vi "Add_Update_Values_sub.vi"(5 "Raw data Filename column name":string, 6 "Edit all Rows?":bool, 7 "Value  Constant?":bool, 8 "Selected Rows":i32[](array[numeric]), 9 "New Values In":string[][](array[string]), 10 "New Chs In":string[](array[string])=[""], 11 "Filename":path) -> (1 "Edit Info":string[][](array[string]))   [LabVIEW 2021]
uses:
  Globals/Constants_global.vi
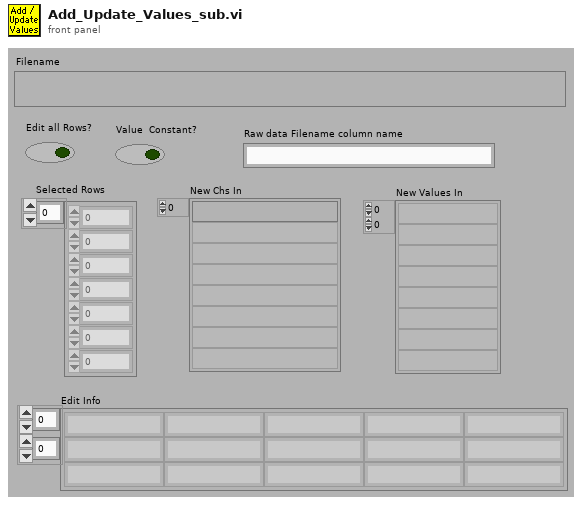
[diagram p1: front panel]
types:
  T1 = enum16{"read/write", "read-only", "write-only", "write-only (truncate)"}
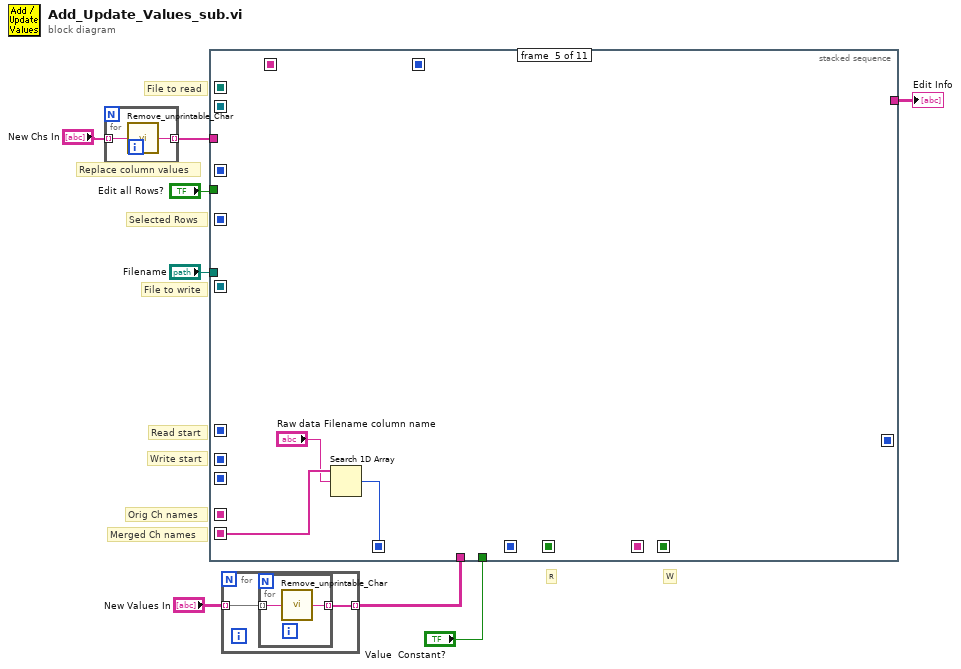
[diagram p0: block diagram]
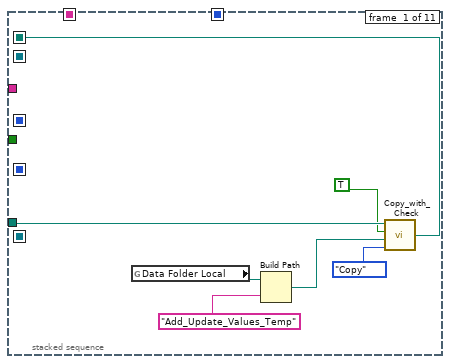
[diagram p2: hidden frame]
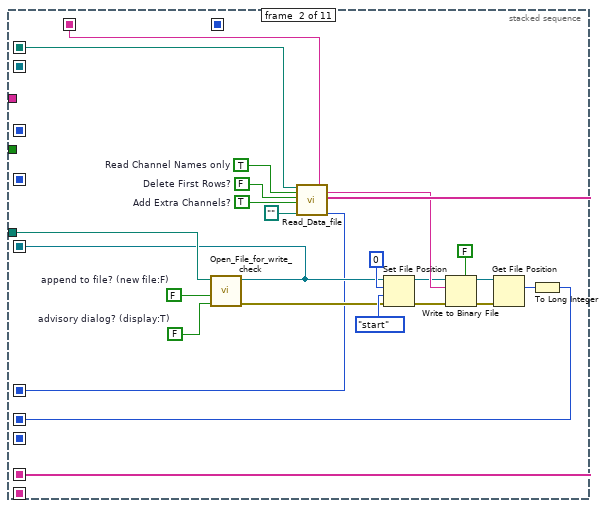
[diagram p3: hidden frame]
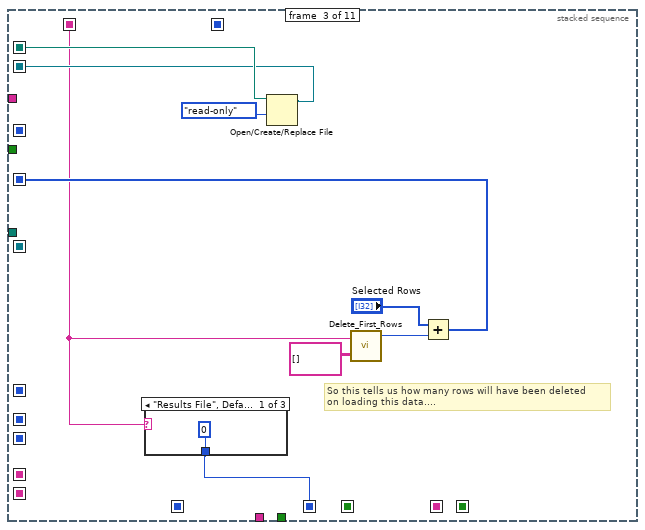
[diagram p4: hidden frame]
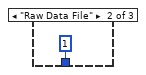
[diagram p5: hidden frame]
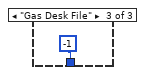
[diagram p6: hidden frame]
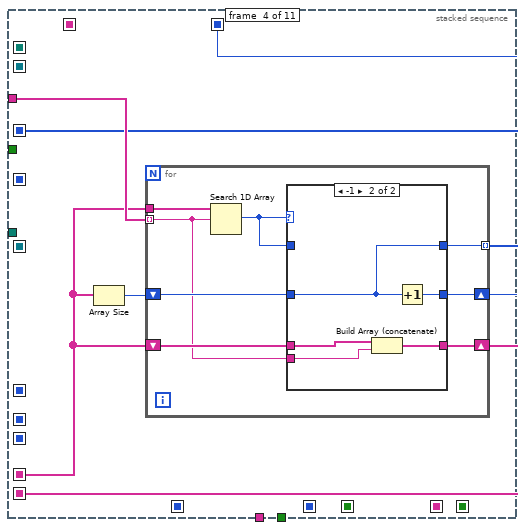
[diagram p7: hidden frame]
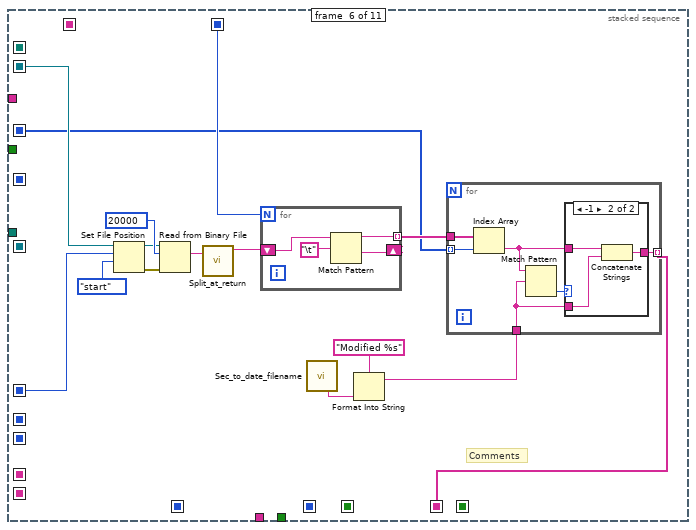
[diagram p9: hidden frame]
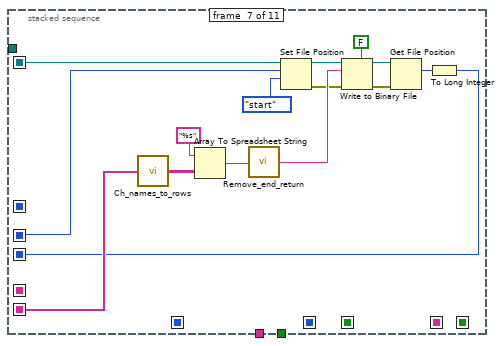
[diagram p11: hidden frame]
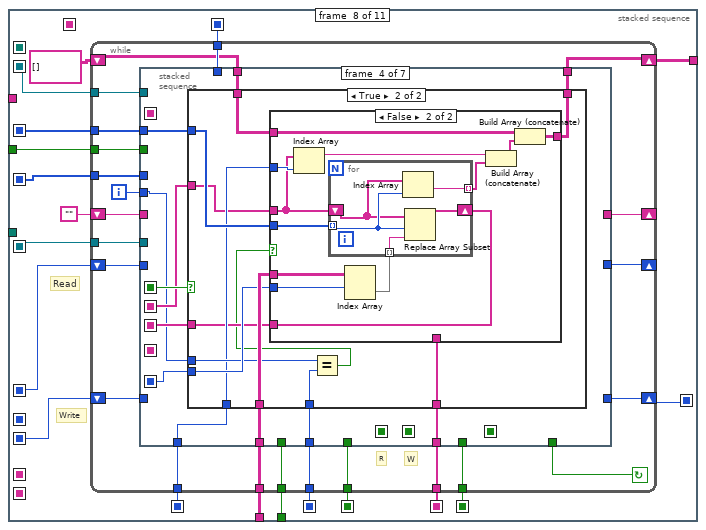
[diagram p12: hidden frame]
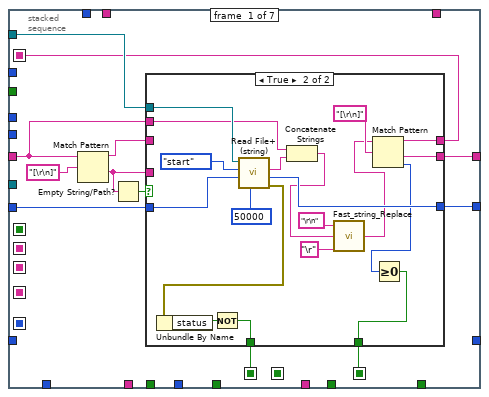
[diagram p13: hidden frame]
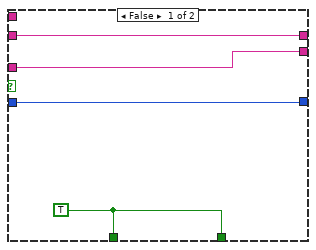
[diagram p14: hidden frame]
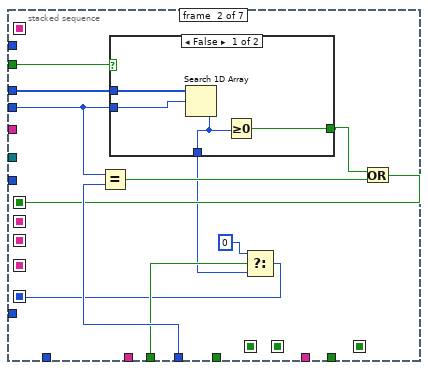
[diagram p15: hidden frame]
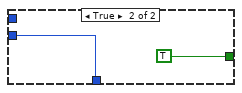
[diagram p16: hidden frame]
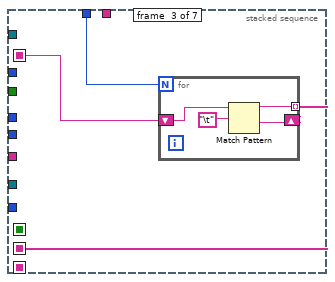
[diagram p17: hidden frame]
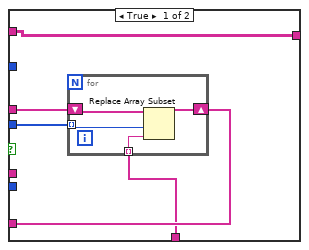
[diagram p19: hidden frame]
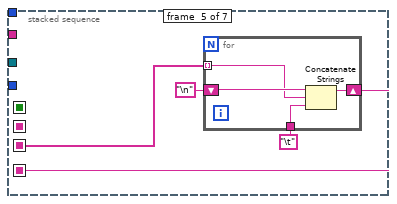
[diagram p20: hidden frame]
diagram:
  # "File to read"
  # "File to write"
  # "Merged Ch names"
  # "Orig Ch names"
  # "Replace column values"
  # "Selected Rows"
  # "Read start"
  # "Write start"
  # "W"
  # "R"
  n1 = for {
    tunnel: "New Chs In" -> [w10] mode=indexing
    tunnel: [w9] -> w4 mode=indexing
    n2 = call "Remove_unprintable_Char.vi"("Input String"=w10) -> ("Output String"=w9:string)
  }
  n3 = for {
    tunnel: "New Values In" -> [w12] mode=indexing
    tunnel: [w11] -> w2 mode=indexing
    n4 = for {
      tunnel: w12 -> [w14] mode=indexing
      tunnel: [w13] -> w11 mode=indexing
      n5 = call "Remove_unprintable_Char.vi"("Input String"=w14) -> ("Output String"=w13:string)
    }
  }
  n6 = stacked-sequence {
    seq-local: [_ _ w48 _ _ _ _ _ _ _ _] -> [_ _ _ _ _ w94 _ w137 _ w314 _]
    seq-local: [_ w31 _ _ _ _ _ _ _ _ _] -> [_ _ _ _ _ w93 _ w139 _ _ _]
    seq-local: [_ _ _ _ _ _ _ w143 _ _ _] -> [_ _ _ _ _ _ _ _ _ _ w318]
    seq-local: [_ _ _ _ _ _ _ w142 _ _ _] -> [_ _ _ _ _ _ _ _ _ _ w320]
    seq-local: [_ _ _ _ _ _ _ w141 _ _ _] -> [_ _ _ _ _ _ _ _ w311 _ _]
    seq-local: [_ _ w51 _ _ _ _ _ _ _ _] -> [_ _ _ _ _ _ _ w140 _ _ _]
    seq-local: [_ w32 _ _ _ _ _ _ _ _ _] -> [_ _ _ _ _ _ w119 _ _ _ _]
    seq-local: [_ w42 _ _ _ _ _ _ _ _ _] -> [_ _ _ w59 _ _ _ _ _ _ _]
    seq-local: [_ _ _ w60 _ _ _ _ _ _ _] -> [_ _ _ _ _ w88 _ w135 _ _ _]
    seq-local: [_ w34 _ _ _ _ _ _ _ _ _] -> [_ _ _ _ _ _ w120 w138 w309 w312 _]
    seq-local: [_ _ _ w58 _ _ _ _ _ _ _] -> [_ _ _ _ _ w96 _ w136 _ _ _]
    seq-local: [_ _ _ w57 _ _ _ _ _ _ _] -> [_ _ _ _ w81 _ w123 _ _ _ _]
    seq-local: [w16 _ _ _ _ _ _ _ _ _ _] -> [_ w41 w49 _ _ _ _ _ _ _ w316]
    seq-local: [_ _ _ _ _ _ w118 _ _ _ _] -> [_ _ _ _ _ _ _ w134 _ _ _]
    seq-local: [_ w30 _ _ _ _ _ _ _ _ _] -> [_ _ w46 _ _ _ _ _ _ _ _]
    seq-local: [_ _ _ _ _ w85 _ _ _ _ _] -> [_ _ _ _ _ _ _ w129 _ _ _]
    seq-local: [_ _ w47 _ _ _ _ _ _ _ _] -> [_ _ _ _ _ _ _ w130 _ _ _]
    seq-local: [_ _ _ _ w80 _ _ _ _ _ _] -> [_ _ _ _ _ _ _ w128 _ _ _]
    tunnel: "Filename" -> [w18 w35 _ _ _ _ _ _ _ _ w317]
    tunnel: w4 -> [_ _ _ w62 _ _ _ _ _ _ _]
    tunnel: "Edit all Rows?" -> [_ _ _ _ _ _ _ w133 _ _ _]
    tunnel: w2 -> [_ _ _ _ _ _ _ w132 _ _ _]
    tunnel: "Value  Constant?" -> [_ _ _ _ _ _ _ w131 _ _ _]
    tunnel: [_ _ _ _ _ _ _ w126 _ _ _] -> w5
    frame #0 {
      n7 = global read "Constants_global.vi" "Data Folder Local"() -> (w20:path)
      n8 = Build Path(base path=w20, name or relative path="Add_Update_Values_Temp") -> (appended path=w19:path)
      n9 = call "Copy_with_Check.vi"("Mode"=enum16{"Move", "Copy"}."Copy", "Target Path"=w19, "Variable Target?"=TRUE, "Source Path"=w18) -> ("Pathname Out"=w16:path)
    }
    frame #1 {
      w22 = FALSE  # Delete First Rows?
      w23 = TRUE  # Add Extra Channels?
      w39 = FALSE  # advisory dialog? (display:T)
      w40 = FALSE  # append to file? (new file:F)
      w43 = TRUE  # Read Channel Names only
      n10 = call "Open_File_for_write_check.vi"("advisory dialog? (display:T)"=w39, "append to file? (new file:F)"=w40, "file path"=w35) -> ("error out"=w36:errorcluster, "refnum"=w34:refnum<file>)  [unwired: 7 out]
      n11 = call "Read_Data_file.vi"("Results file"=w41, "Read Channel Names only"=w43, "Delete First Rows?"=w22, "Add Extra Channels?"=w23, "Template File"=path "") -> ("Filetype"=w30:string, "String Before"=w33:string, "Ch names Out"=w42:string[], "Start Bytes"=w31:i32)  [unwired: 2 in, 9 out]
      n12 = Set File Position(offset (in bytes) (0)=0 ("pos offset (0)"), refnum=w34, from (0:start)=enum16{"start", "end", "current"}."start" ("pos mode (0:2)"), error in=w36) -> (refnum out=w29:refnum<file>, error out=w28:errorcluster)
      n13 = Write to Binary File(file (use dialog)=w29, data=w33, error in=w28, 5:FALSE ("prepend array or string size? (T)")) -> (refnum out=w27:refnum<file>, error out=w26:errorcluster)  [unwired: 3 out]
      n14 = Get File Position(4:w26, 7:w27) -> (2:w25:i64)  [unwired: 2 out]
      n15 = To Long Integer(number=w25) -> (32bit integer=w32:i32)
    }
    frame #2 {
      # "So this tells us how many rows will have been deleted\non loading this data...."
      n16 = case shown="\"Results File\", Default" w46 {
        tunnel: [0 ("Comments Row Number") 1 ("Comments Row Number") -1 ("Comments Row Number")] -> w47
        frame "Results File", Default {
        }
        frame "Raw Data File" {
        }
        frame "Gas Desk File" {
        }
      }
      n17 = Open/Create/Replace File(file path (use dialog)=w49, access (0:read/write)=T1."read-only" ("open mode (0)")) -> (refnum out=w48:refnum<file>)  [unwired: 1 in, 5 out]
      n18 = call "Delete_First_Rows.vi"("File Type"=w46, "Data In"=string[][] []) -> ("Rows removed"=w53:i32)  [unwired: 2 out]
      n19 = Add(x="Selected Rows", y=w53) -> (x+y=w51:i32[])
    }
    frame #3 {
      n20 = Array Size(array=w59) -> (size(s)=w61:i32)
      n21 = for {
        tunnel: w59 -> [w70]
        tunnel: w62 -> [w63] mode=indexing
        shift-right: [w69] -> w58
        shift-left: w61 -> [w68]
        tunnel: [w67] -> w60 mode=indexing
        shift-right: [w64] -> w57
        shift-left: w59 -> [w65]
        n22 = Search 1D Array(1D array=w70, element=w63) -> (index of element=w66:i32)  [unwired: 1 out]
        n23 = case shown="-1" w66 {
          tunnel: [w72 w78] -> w69
          tunnel: w68 -> [w72 w77]
          tunnel: [w73 w77] -> w67
          tunnel: w66 -> [w73 _]
          tunnel: w65 -> [w71 w76]
          tunnel: [w71 w75] -> w64
          tunnel: w63 -> [_ w74]
          frame 0, Default {
          }
          frame -1 {
            n24 = Build Array (concatenate)(w76, w74) -> (w75:string[])
            n25 = Increment(x=w77) -> (x+1=w78:i32)
          }
        }
      }
    }
    frame #4 {
      n26 = Search 1D Array(1D array=w81, element="Raw data Filename column name") -> (index of element=w80:i32)  [unwired: 1 out]
    }
    frame #5 {
      # "Comments"
      n27 = Set File Position(offset (in bytes) (0)=w93, refnum=w94, from (0:start)=enum16{"start", "end", "current"}."start" ("pos mode (rel. to current:2)")) -> (refnum out=w84:refnum<file>, error out=w83:errorcluster)  [unwired: 1 in]
      n28 = Read from Binary File(8:w83, 10:20000 ("count"), 11:w84) -> (2:w91:string)  [unwired: 6 out]
      n29 = call "Split_at_return.vi"("String"=w91) -> ("before substring"=w90:string)  [unwired: 1 in, 3 out]
      n30 = for {
        N: w96 -> [_]
        shift-right: [w108] -> _
        shift-left: w90 -> [w109]
        tunnel: [w107] -> w89 mode=indexing
        n31 = Match Pattern(string=w109, regular expression="\t") -> (before substring=w107:string, after substring=w108:string)  [unwired: 3 out]
      }
      n32 = call "Sec_to_date_filename.vi"() -> ("YYYY-mm-DD HH:MM"=w82:string)  [unwired: 6 in, 9 out]
      n33 = Format Into String(format string="Modified %s" ("Format String"), w82) -> (resulting string=w86:string)  [unwired: 2 in, 1 out]
      n34 = for {
        tunnel: w89 -> [w102]
        tunnel: w88 -> [w101] mode=indexing
        tunnel: w86 -> [w99]
        tunnel: [w100] -> w85 mode=indexing
        n35 = Index Array(array=w102, index=w101) -> (element=w98:string)
        n36 = Match Pattern(string=w98, regular expression=w99) -> (offset past match=w97:i32)  [unwired: 4 out]
        n37 = case shown="-1" w97 {
          tunnel: w98 -> [w103 w106]
          tunnel: w99 -> [_ w105]
          tunnel: [w103 w104] -> w100
          frame 0, Default {
          }
          frame -1 {
            n38 = Concatenate Strings(w106, w105) -> (w104:string)
          }
        }
      }
    }
    frame #6 {
      n39 = call "Ch_names_to_rows.vi"("Channel Names"=w123) -> ("3 Row names"=w124:string[][])
      n40 = Array To Spreadsheet String(array=w124, 3:"%s" ("format string")) -> (spreadsheet string=w122:string)  [unwired: 1 out]
      n41 = call "Remove_end_return.vi"("Input string"=w122) -> ("Output string"=w117:string)
      n42 = Set File Position(offset (in bytes) (0)=w119, refnum=w120, from (0:start)=enum16{"start", "end", "current"}."start" ("pos mode (0:2)")) -> (refnum out=w116:refnum<file>, error out=w115:errorcluster)  [unwired: 1 in]
      n43 = Write to Binary File(file (use dialog)=w116, data=w117, error in=w115, 5:FALSE ("prepend array or string size? (T)")) -> (refnum out=w114:refnum<file>, error out=w113:errorcluster)  [unwired: 3 out]
      n44 = Get File Position(4:w113, 7:w114) -> (2:w112:i64)  [unwired: 2 out]
      n45 = To Long Integer(number=w112) -> (32bit integer=w118:i32)
    }
    frame #7 {
      # "Write"
      # "Read"
      n46 = while {
        tunnel: [w158] -> w142
        tunnel: [w159] -> w143
        shift-left: w134 -> [w162]
        shift-right: [w161] -> w141
        tunnel: w137 -> [w164]
        shift-left: w139 -> [w166]
        shift-right: [w165] -> _
        shift-left: "" -> [w167]
        shift-right: [w163] -> _
        tunnel: w140 -> [w157]
        tunnel: w138 -> [w155]
        tunnel: w136 -> [w154]
        tunnel: w133 -> [w153]
        tunnel: w135 -> [w152]
        tunnel: w132 -> [w151]
        tunnel: w131 -> [w150]
        tunnel: w130 -> [w149]
        tunnel: w129 -> [w148]
        tunnel: w128 -> [w147]
        shift-right: [w145] -> w126
        shift-left: string[][] [] -> [w146]
        i -> [w156]
        stop <- w160 continue-if-true
        # "R"
        # "W"
        n47 = stacked-sequence {
          seq-local: [w173 _ _ _ _ _ _] -> [_ _ w221 _ _ _ _]
          seq-local: [_ _ _ _ _ w299 _] -> [_ _ _ _ _ _ w302]
          seq-local: [w174 _ _ _ _ _ _] -> [_ _ _ _ _ _ w304]
          seq-local: [w175 _ _ _ _ _ _] -> [_ _ _ _ _ _ w303]
          seq-local: [_ w208 _ _ _ _ _] -> [_ _ _ w237 _ _ _]
          seq-local: [_ _ _ _ w282 _ _] -> [_ _ _ _ _ w298 _]
          seq-local: [_ _ w220 _ _ _ _] -> [_ _ _ w235 _ _ _]
          seq-local: [_ _ _ w234 _ _ _] -> [_ _ _ _ w279 _ _]
          seq-local: [_ w203 _ _ _ _ _] -> [_ _ _ w227 _ _ _]
          tunnel: w167 -> [w171 _ _ _ _ _ _]
          tunnel: w166 -> [w179 _ _ _ _ _ _]
          tunnel: [w178 _ _ _ _ _ _] -> w165
          tunnel: w164 -> [w177 _ _ _ _ _ _]
          tunnel: [w176 _ _ _ _ _ _] -> w163
          tunnel: w162 -> [_ _ _ _ _ w301 _]
          tunnel: [_ _ _ _ _ w300 _] -> w161
          tunnel: [_ _ _ _ _ _ w305] -> w160
          tunnel: [_ _ _ _ _ _ w303] -> w159
          tunnel: [_ _ _ _ _ _ w302] -> w158
          tunnel: w157 -> [_ w213 _ _ _ _ _]
          tunnel: w156 -> [_ w210 _ w232 _ _ _]
          tunnel: w155 -> [_ _ _ _ _ w297 _]
          tunnel: w154 -> [_ _ w222 _ _ _ _]
          tunnel: w153 -> [_ w212 _ _ _ _ _]
          tunnel: w152 -> [_ _ _ w238 _ _ _]
          tunnel: w151 -> [_ _ _ w236 _ _ _]
          tunnel: w150 -> [_ w206 _ _ _ _ _]
          tunnel: w149 -> [_ w211 _ w233 _ _ _]
          tunnel: w148 -> [_ _ _ w231 _ _ _]
          tunnel: w147 -> [_ _ _ w230 _ _ _]
          tunnel: w146 -> [_ _ _ w229 _ _ _]
          tunnel: [_ _ _ w228 _ _ _] -> w145
          frame #0 {
            n48 = Match Pattern(string=w171, regular expression="[\r\n]") -> (before substring=w170:string, after substring=w168:string)  [unwired: 3 out]
            n49 = Empty String/Path?(string/path=w168) -> (empty?=w169:bool)
            n50 = case shown="True" w169 {
              tunnel: w179 -> [w183 w202]
              tunnel: [w183 w200] -> w178
              tunnel: w177 -> [_ w199]
              tunnel: w171 -> [_ w198]
              tunnel: [w182 w190] -> w176
              tunnel: w168 -> [w182 _]
              tunnel: [w181 w195] -> w175
              tunnel: [w181 w187] -> w174
              tunnel: [w180 w189] -> w173
              tunnel: w170 -> [w180 _]
              frame False {
                w181 = TRUE
              }
              frame True {
                n51 = call <vilib>:"Read File+ (string).vi"("count"=50000, "pos offset (bytes:0)"=w202, "pos mode (rel. to current:2)"=enum16{"start", "end", "current"}."start", "refnum"=w199) -> ("error out"=w197:errorcluster, "mark after read (bytes)"=w200:i32, "string"=w186:string)  [unwired: 1 in, 4 out]
                n52 = Unbundle By Name(w197) -> ("status"=w196:bool)
                n53 = Not(x=w196) -> (.not. x?=w195:bool)
                n54 = Concatenate Strings(w198, w186) -> (w185:string)
                n55 = call "Fast_string_Replace.vi"("Replace match with:"="\r" ("regular expression"), "Input String"=w185, "regular expression"="\r\n") -> ("Output String"=w184:string)  [unwired: 2 out]
                n56 = Match Pattern(string=w184, regular expression="[\r\n]") -> (before substring=w189:string, after substring=w190:string, offset past match=w188:i32)  [unwired: 2 out]
                n57 = Greater Or Equal To 0?(x=w188) -> (x >= 0?=w187:bool)
              }
            }
          }
          frame #1 {
            n58 = Equal?(x=w210, y=w211) -> (x = y?=w209:bool)
            n59 = case shown="False" w212 {
              tunnel: w213 -> [w217 _]
              tunnel: w210 -> [w216 w218]
              tunnel: [w215 TRUE] -> w207
              tunnel: [w214 w218] -> w205
              frame False {
                n60 = Search 1D Array(1D array=w217, element=w216) -> (index of element=w214:i32)  [unwired: 1 out]
                n61 = Greater Or Equal To 0?(x=w214) -> (x >= 0?=w215:bool)
              }
              frame True {
              }
            }
            n62 = Select(t=0, s=w206, f=w205) -> (s? t:f=w203:i32)
            n63 = Or(x=w207, y=w209) -> (x .or. y?=w208:bool)
          }
          frame #2 {
            n64 = for {
              N: w222 -> [_]
              shift-right: [w224] -> _
              shift-left: w221 -> [w225]
              tunnel: [w223] -> w220 mode=indexing
              n65 = Match Pattern(string=w225, regular expression="\t") -> (before substring=w223:string, after substring=w224:string)  [unwired: 3 out]
            }
          }
          frame #3 {
            n66 = case shown="True" w237 {
              tunnel: w238 -> [_ w252]
              tunnel: w236 -> [_ w251]
              tunnel: w235 -> [w240 w245]
              tunnel: w227 -> [_ w250]
              tunnel: [w240 w246] -> w234
              tunnel: w233 -> [_ w249]
              tunnel: w232 -> [_ w248]
              tunnel: w231 -> [_ w241]
              tunnel: w230 -> [_ w247]
              tunnel: w229 -> [w239 w244]
              tunnel: [w239 w243] -> w228
              frame False {
              }
              frame True {
                n67 = Equal?(x=w248, y=w249) -> (x = y?=w242:bool)
                n68 = case shown="False" w242 {
                  tunnel: w252 -> [w257 w273]
                  tunnel: w251 -> [_ w272]
                  tunnel: w250 -> [_ w271]
                  tunnel: w247 -> [_ w269]
                  tunnel: [w256 w268] -> w246
                  tunnel: w245 -> [w255 w262]
                  tunnel: w244 -> [w253 w267]
                  tunnel: [w253 w266] -> w243
                  tunnel: w241 -> [w254 _]
                  frame True {
                    n69 = for {
                      shift-right: [w261] -> w256
                      shift-left: w255 -> [w259]
                      tunnel: w257 -> [w260] mode=indexing
                      tunnel: w254 -> [w258] mode=indexing
                      n70 = Replace Array Subset(array=w259, new element=w258, index=w260) -> (w261:string[])
                    }
                  }
                  frame False {
                    n71 = Index Array(array=w262, index=w269) -> (element=w264:string)
                    n72 = Index Array(array=w272, index (row)=w271) -> (element=w270:string[])  [unwired: 1 in]
                    n73 = for {
                      shift-right: [w278] -> w268
                      shift-left: w262 -> [w276]
                      tunnel: w273 -> [w277] mode=indexing
                      tunnel: w270 -> [w275] mode=indexing
                      tunnel: [w274] -> w265 mode=indexing
                      n74 = Index Array(array=w276, index=w277) -> (element=w274:string)
                      n75 = Replace Array Subset(array=w276, new element=w275, index=w277) -> (w278:string[])
                    }
                    n76 = Build Array (concatenate)(w264, w265) -> (w263:string[])
                    n77 = Build Array (concatenate)(w267, w263) -> (w266:string[][])
                  }
                }
              }
            }
          }
          frame #4 {
            n78 = for {
              tunnel: w279 -> [w283] mode=indexing
              shift-right: [w284] -> w282
              shift-left: "\n" -> [w286]
              tunnel: "\t" -> [w285]
              n79 = Concatenate Strings(w286, w283, w285) -> (w284:string)
            }
          }
          frame #5 {
            n80 = Set File Position(offset (in bytes) (0)=w301, refnum=w297, from (0:start)=enum16{"start", "end", "current"}."start" ("pos mode (0:2)")) -> (refnum out=w292:refnum<file>, error out=w291:errorcluster)  [unwired: 1 in]
            n81 = Write to Binary File(file (use dialog)=w292, data=w298, error in=w291, 5:FALSE ("prepend array or string size? (T)")) -> (refnum out=w290:refnum<file>, error out=w289:errorcluster)  [unwired: 3 out]
            n82 = Get File Position(4:w289, 7:w290) -> (0:w293:errorcluster, 2:w288:i64)  [unwired: 1 out]
            n83 = Unbundle By Name(w293) -> ("status"=w294:bool)
            n84 = To Long Integer(number=w288) -> (32bit integer=w296:i32)
            n85 = Decrement(x=w296) -> (x-1=w300:i32)
            n86 = Not(x=w294) -> (.not. x?=w299:bool)
          }
          frame #6 {
            n87 = Compound Arithmetic op=AND(w303, w302, w304) -> (w305:bool)
          }
        }
      }
    }
    frame #8 {
      n88 = call <vilib>:"compatCalcOffset.vi"("pos offset (0)"=w311, "pos mode (0:1)"=enum16{"start", "end", "current"}."start", "refnum"=w309) -> ("error out"=w308:errorcluster, "offset"=w307:i32, "dup refnum"=w306:refnum<file>)  [unwired: 1 in, 5 out]
      n89 = Set File Size(4:w308, 6:w307, 7:w306) -> ()  [unwired: 2 out]
    }
    frame #9 {
      n90 = Build Array(w314, w312) -> (w313:refnum<file>[])
      n91 = for {
        tunnel: w313 -> [w315] mode=indexing
        n92 = Close File(refnum=w315) -> ()  [unwired: 1 in, 2 out]
      }
    }
    frame #10 {
      n93 = Not And(1:w320, 2:w318) -> (0:w319:bool)
      n94 = case shown="True" w319 {
        tunnel: w316 -> [_ w323]
        tunnel: w317 -> [_ w322]
        frame False {
        }
        frame True {
          w327 = TRUE  # Dialog Box
          n95 = Format Into String(format string="whilst reading from file %s\nand writing to file %s", w323, w322) -> (resulting string=w321:string)  [unwired: 2 in, 1 out]
          n96 = Bundle By Name(cluster=errorcluster {"status"=FALSE, "code"=0, "source"=""} ("error in (no error)"), "status"=TRUE ("Bundle Element"), "source"=w321) -> (w328:errorcluster)
          n97 = call "EnFlo_Error_Handler.vi"("error in (no error)"=w328, "Error Type"="File Rewrite Error", "Dialog Box (F)"=w327) -> ()  [unwired: 3 out]
        }
      }
    }
  }
  "Edit Info" <- w5
